vi "Peak_removal.vi"(10 "tolerance (Deviation)":dbl=3.0, 11 "Input Waveform":waveform(dbl)(graph)) -> (2 "Tolerance Level":dbl, 3 "Peaks Removed":waveform(dbl)(graph))   [LabVIEW 2015]
uses:
  <vilib>/Analysis/NI_AALBase.lvlib
panel:
  out "standard deviation":dbl format="%0.2f"
  out "mean":dbl format="%0.2f"
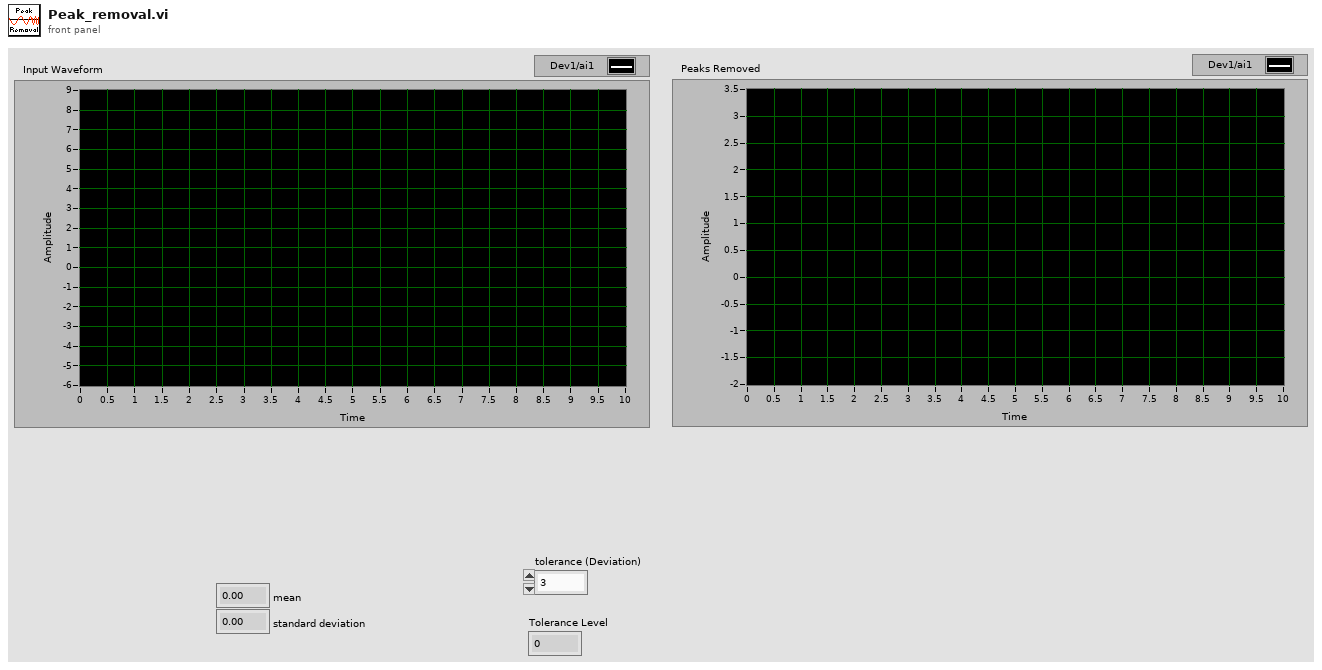
[diagram p1: front panel]
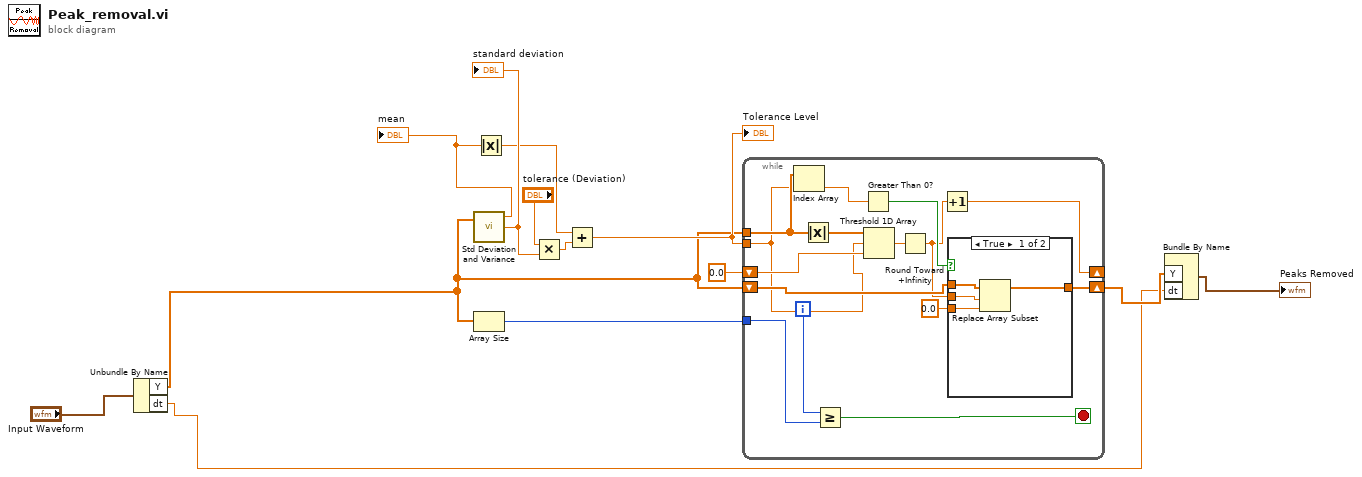
[diagram p0: block diagram]
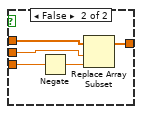
[diagram p2: hidden frame]
diagram:
  n1 = Unbundle By Name("Input Waveform") -> ("Y"=w5:dbl[], "dt"=w2:dbl)
  n2 = call <vilib>:"Std Deviation and Variance.vi"("X"=w5) -> ("mean"=w7:dbl, "standard deviation"=w13:dbl)  [unwired: 1 in, 1 out]
  "mean" <- w7
  "standard deviation" <- w13
  n3 = Array Size(array=w5) -> (size(s)=w9:i32)
  n4 = Absolute Value(x=w7) -> (abs(x)=w6:dbl)
  n5 = Multiply(x="tolerance (Deviation)", y=w13) -> (x*y=w11:dbl)
  n6 = Add(x=w6, y=w11) -> (x+y=w10:dbl)
  "Tolerance Level" <- w10
  n7 = while {
    tunnel: w5 -> [w21]
    tunnel: w10 -> [w15]
    shift-right: [w25] -> _
    shift-left: 0.0 -> [w20]
    shift-right: [w27] -> w3
    shift-left: w5 -> [w17]
    tunnel: w9 -> [w23]
    i -> [w24]
    stop <- w26 stop-if-true
    n8 = Index Array(array=w21, index=w15) -> (element=w19:dbl)
    n9 = Absolute Value(x=w21) -> (abs(x)=w22:dbl[])
    n10 = Greater Or Equal?(x=w24, y=w23) -> (x >= y?=w26:bool)
    n11 = Greater Than 0?(x=w19) -> (x > 0?=w18:bool)
    n12 = Threshold 1D Array(1:w20, 2:w15, 3:w22) -> (0:w28:dbl)
    n13 = Round Toward +Infinity(x=w28) -> (ceil(x): smallest int >= x=w16:dbl)
    n14 = Increment(x=w16) -> (x+1=w25:dbl)
    n15 = case shown="True" w18 {
      tunnel: [w32 w37] -> w27
      tunnel: w17 -> [w31 w36]
      tunnel: w16 -> [w30 w35]
      tunnel: 0.0 -> [w29 w33]
      frame True {
        n16 = Replace Array Subset(array=w31, new element=w29, index=w30) -> (w32:dbl[])
      }
      frame False {
        n17 = Negate(x=w33) -> (-x=w34:dbl)
        n18 = Replace Array Subset(array=w36, new element=w34, index=w35) -> (w37:dbl[])
      }
    }
  }
  n19 = Bundle By Name("Y"=w3, "dt"=w2) -> (→"Peaks Removed":waveform(dbl))  [unwired: 1 in]
